vi "getPacketType.vi"(11 "read buffer":string) -> (3 "type":i8)   [LabVIEW 2011]
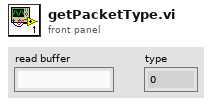
[diagram p1: front panel]
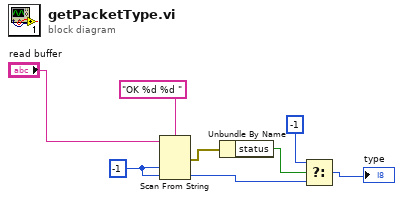
[diagram p0: block diagram]
diagram:
  w6 = i8 -1 ("default value 1")
  n1 = Scan From String(format string="OK %d %d ", input string="read buffer", default 1=w6, default 2=w6) -> (error out=w5:errorcluster, output 2=w2:i8)  [unwired: 3 in, 2 out]
  n2 = Unbundle By Name(w5) -> ("status"=w4:bool)
  n3 = Select(t=i8 -1 ("default value 1"), s=w4, f=w2) -> (s? t:f=→"type":i8)
